vi "EventLog.Buffer.vi"(7 "action (get)":T7=enum."get", 8 "error in":errorcluster, 9 "Event.Sets":T5 {"dtm_End" format="%<%.1X\n%x>T"; "dtm_Begin" format="%<%.1X\n%x>T"}, 10 "Event in":T1={"ts"=0.0, "lev"=enum."Debug", "src"=enum."All", "msg"=enum."Log out", "arg"=[], "msg_str"=""} {"ts" format="%<%X\n%x>T"}, 11 "Translations":string[](array[string])) -> (0 "error out":errorcluster, 1 "Translated Msg":string, 2 "data out":T1[](array[typedef]) {"ts" format="%<%X\n%x>T"}, 3 "Event out":T1={"ts"=0.0, "lev"=enum."Debug", "src"=enum."All", "msg"=enum."Log out", "arg"=[], "msg_str"=""} {"ts" format="%<%X\n%x>T"})   [LabVIEW 2016]
uses:
  EventLog.Buffer.Action.ctl
  EventLog.EventGui.ctl
  EventLog.EventLevel.ctl
  EventLog.EventSource.ctl
  Translator/Translator.Message.ctl
  EventLog.Gui.Sets.ctl
  EventLog.EventLevelOperatorGui.ctl
panel:
  out "Translations out":string[](array[string])
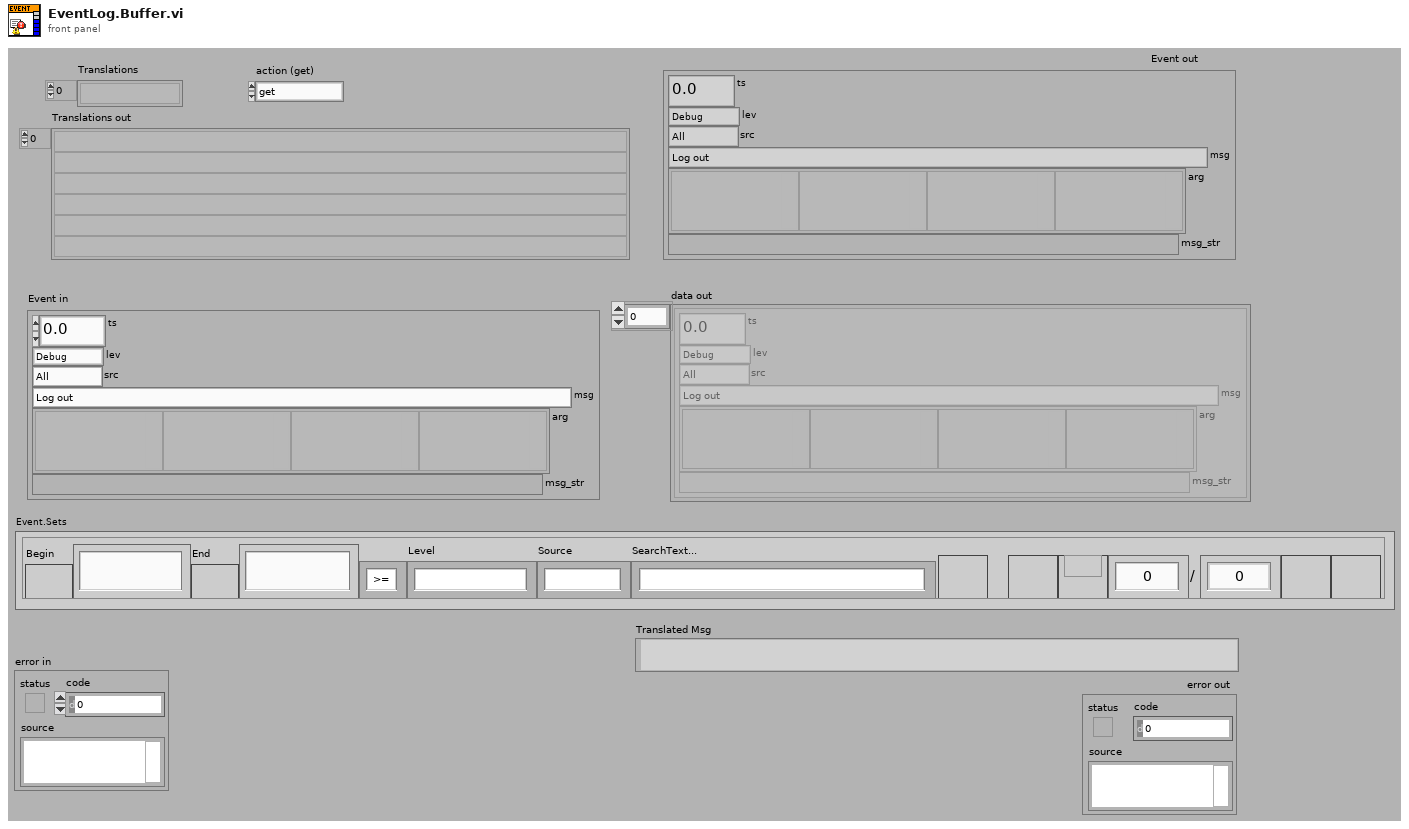
[diagram p1: front panel]
types:
  T1 = typedef "EventLog.EventGui.ctl" = cluster{"ts":dbl, "lev":T2, "src":T3, "msg":T4, "arg":variant[], "msg_str":string}
  T2 = typedef "EventLog.EventLevel.ctl" = enum8{"Debug", "Info", "Warning", "Error"}
  T3 = typedef "EventLog.EventSource.ctl" = enum16{"All", "Gui", "Cache", "PLC1", "PLC2", "PLC3", "DB", "DB01", "DB02", "DB03", "DB04", "DB05", "DB06", "DB07", "DB08", "DB09", "DB10", "DB11", "DB12", "DB13", "DB14", "DB15", "DB16"}
  T4 = typedef "Translator.Message.ctl" = enum16{"-", "Event confirmed", "Log out", "Log in", "Shutdown", "Cancel", "Start", "Continue", "Stop", "On", "Off", "OK", "NOK", "NOK %s", "This", "Prev", "Home", "Work", "In progress...", "Missing", "Empty", "Hardware failure", "Initial", "Error %d >> %s", "Error %d >> %s >> %s", "Starting %s", "Quitting %s", "Configured", "Initializing", "Quitting", "Loading", "Running %s", "Stopped", "Summary", "Do you want to continue?", "Do you want to exit?", "Log out?", "System", "All", "IDLE", "Translating...%s", "Not found", "Alarm %s", "Run", "Skip", "Abort", "Repeat", "Please wait...", "Database disconnected", "Login to database successful", "Login to database failed: %d; %s", "Get process step data for %s", "Changeover off", "Changeover into %s", "Product %s | %s found in cache with status %d at previous station", "Product %s | %s found in database with status %d at previous station", "Product %s | %s not found in cache at previous station", "Product %s | %s not found in database at previous station", "Product %s | %s found in cache with status %d at this station (%d repetion)", "Product %s | %s found in database with status %d at this station (%d repetition)", "Product %s | %s not found in cache at this station", "Product %s | %s not found in database at this station", "Product %s | %s found in cache for component %s | %s", "Product %s | %s found in database for component %s | %s", "Product not found in cache for component %s | %s", "Product not found in database for component %s | %s", "Product %s | %s connected with component %s | %s (cache)", "Product %s | %s connected with component %s | %s (database)", "New data for %s | %s (cache)", "New data for %s | %s (database)", "File %s moved (cache)", "File %s deleted (cache)", "Msg %d >> %s", "PLC LifeBit Failure", "Reconnecting DB", "Reconnecting PLC", "Free disk space is below 1GB - contact technician", "Unable to check product status"}
  T5 = typedef "EventLog.Gui.Sets.ctl" = cluster{"IncludeBegin":bool, "dtm_Begin":timestamp, "IncludeEnd":bool, "dtm_End":timestamp, "Events Level Operator":T6, "Level":u16, "Source":u16, "SearchText":string, "Refresh":bool, "Pages":i32, "PageNo":i32, "First":bool, "Prev":bool, "Next":bool, "Last":bool}
  T6 = typedef "EventLog.EventLevelOperatorGui.ctl" = enum16{">=", "=", "<="}
  T7 = typedef "EventLog.Buffer.Action.ctl" = enum16{"init", "re-init", "clear", "set translator", "translate", "add", "get"}
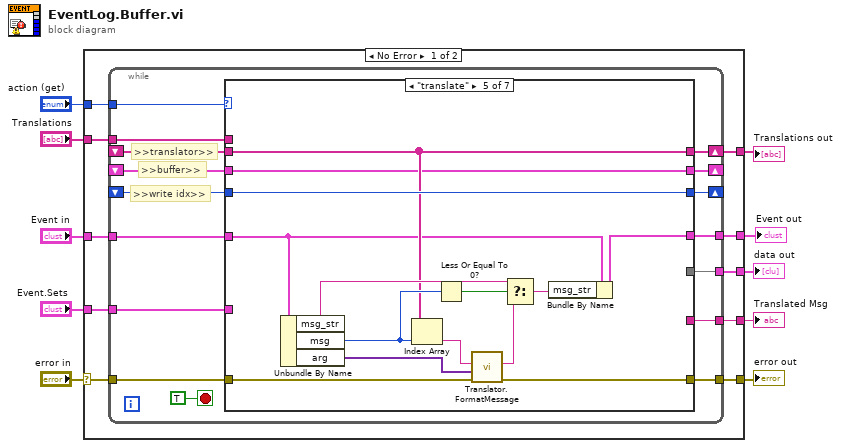
[diagram p0: block diagram]
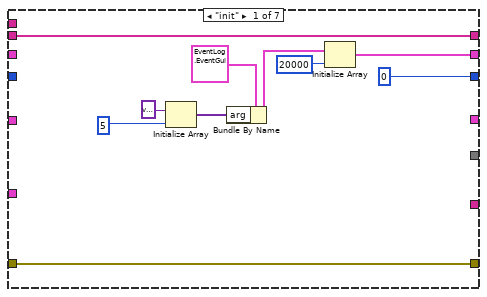
[diagram p2: hidden frame]
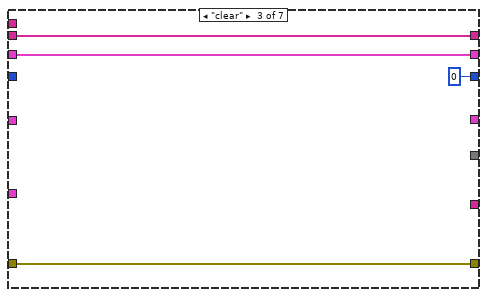
[diagram p4: hidden frame]
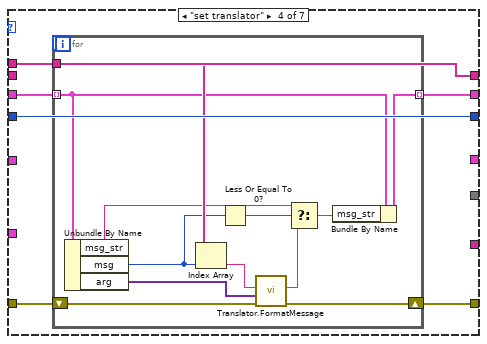
[diagram p5: hidden frame]
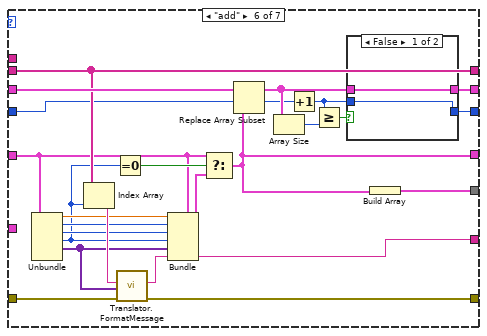
[diagram p6: hidden frame]
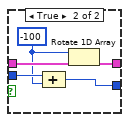
[diagram p7: hidden frame]
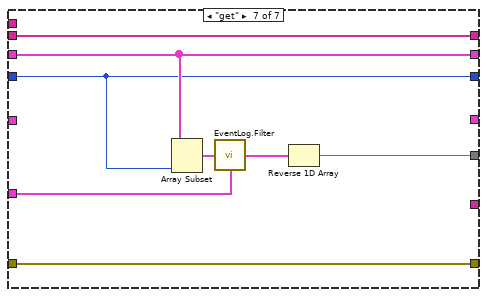
[diagram p8: hidden frame]
diagram:
  n1 = case shown="No Error" "error in" {
    selector: "error in" -> [w14 w125]
    tunnel: "action (get)" -> [w20 _]
    tunnel: "Event in" -> [w19 _]
    tunnel: [w18 _] -> w8
    tunnel: "Event.Sets" -> [w17 _]
    tunnel: "Translations" -> [w16 _]
    tunnel: [w15 w125] -> w6
    tunnel: [w13 _] -> w3
    tunnel: [w12 _] -> w2
    tunnel: [w11 _] -> w1
    frame No Error {
      n2 = while {
        tunnel: w20 -> [w35]
        tunnel: w19 -> [w34]
        shift-right: [w33] -> _
        shift-left: _ -> [w32]
        tunnel: [w31] -> w18
        shift-right: [w30] -> _
        shift-left: _ -> [w29]
        tunnel: w17 -> [w28]
        tunnel: w16 -> [w27]
        shift-right: [w26] -> w13
        shift-left: _ -> [w25]
        tunnel: w14 -> [w24]
        tunnel: [w23] -> w15
        tunnel: [w22] -> w12
        tunnel: [w21] -> w11
        stop <- TRUE stop-if-true
        # ">>write idx>>"
        # ">>translator>>"
        # ">>buffer>>"
        n3 = case shown="\"translate\"" w35 {
          tunnel: w34 -> [_ _ _ _ w74 w96 _]
          tunnel: [w45 w50 w54 w56 w75 w104 w118] -> w33
          tunnel: w32 -> [_ w50 w54 w59 w75 w109 w118]
          tunnel: [_ _ _ _ _ w98 w124] -> w31
          tunnel: [0 w49 0 w60 w86 w103 w117] -> w30
          tunnel: w29 -> [_ w49 _ w60 w86 w99 w117]
          tunnel: w28 -> [_ _ _ _ _ _ w122]
          tunnel: w27 -> [_ _ _ w55 _ _ _]
          tunnel: [w40 w48 w53 w55 w76 w101 w120] -> w26
          tunnel: w25 -> [w40 w48 w53 _ w76 w101 w120]
          tunnel: w24 -> [w38 w47 w52 w57 w84 w102 w119]
          tunnel: [w38 w47 w52 w58 w85 w91 w119] -> w23
          tunnel: [_ _ _ _ _ w87 _] -> w22
          tunnel: [_ _ _ _ w73 w90 _] -> w21
          frame "init" {
            n4 = Initialize Array(variant ("Variant"), 5 ("dimension size")) -> (w41:variant[])
            n5 = Bundle By Name(cluster=T1 {"ts"=0.0, "lev"=enum."Debug", "src"=enum."All", "msg"=enum."Log out", "arg"=[], "msg_str"=""} ("Event (GUI)"), "arg"=w41) -> (w44:T1)
            n6 = Initialize Array(w44, 20000 ("dimension size")) -> (w45:T1[])
          }
          frame "re-init" {
          }
          frame "clear" {
          }
          frame "set translator" {
            n7 = for {
              tunnel: w59 -> [w68] mode=indexing
              tunnel: w55 -> [w69]
              shift-right: [w71] -> w58
              shift-left: w57 -> [w70]
              tunnel: [w67] -> w56 mode=indexing
              n8 = Unbundle By Name(w68) -> ("msg_str"=w64:string, "msg"=w65:T4, "arg"=w72:variant[])
              n9 = Index Array(array=w69, index=w65) -> (element=w66:string)
              n10 = Less Or Equal To 0?(x=w65) -> (x <= 0?=w63:bool)
              n11 = call "Translator.FormatMessage.vi"("error in (no error)"=w70, "Arguments"=w72, "Msg"=w66) -> ("error out"=w71:errorcluster, "Translated Msg"=w62:string)  [unwired: 7 in]
              n12 = Select(t=w64, s=w63, f=w62) -> (s? t:f=w61:string)
              n13 = Bundle By Name(cluster=w68, "msg_str"=w61) -> (w67:T1)
            }
          }
          frame "translate" {
            n14 = Unbundle By Name(w74) -> ("msg_str"=w80:string, "msg"=w81:T4, "arg"=w83:variant[])
            n15 = Index Array(array=w76, index=w81) -> (element=w82:string)
            n16 = Less Or Equal To 0?(x=w81) -> (x <= 0?=w79:bool)
            n17 = call "Translator.FormatMessage.vi"("error in (no error)"=w84, "Arguments"=w83, "Msg"=w82) -> ("error out"=w85:errorcluster, "Translated Msg"=w78:string)  [unwired: 7 in]
            n18 = Select(t=w80, s=w79, f=w78) -> (s? t:f=w77:string)
            n19 = Bundle By Name(cluster=w74, "msg_str"=w77) -> (w73:T1)
          }
          frame "add" {
            n20 = Unbundle(w96) -> ("ts"=w94:dbl, "lev"=w93:T2, "src"=w92:T3, "msg"=w89:T4, "arg"=w88:variant[])  [unwired: 1 out]
            n21 = Index Array(array=w101, index=w89) -> (element=w100:string)
            n22 = Equal To 0?(x=w89) -> (x = 0?=w97:bool)
            n23 = call "Translator.FormatMessage.vi"("error in (no error)"=w102, "Arguments"=w88, "Msg"=w100) -> ("error out"=w91:errorcluster, "Translated Msg"=w87:string)  [unwired: 7 in]
            n24 = Bundle(cluster=w96, "ts"=w94, "lev"=w93, "src"=w92, "msg"=w89, "arg"=w88, "msg_str"=w87) -> (w95:T1)
            n25 = Select(t=w96, s=w97, f=w95) -> (s? t:f=w90:T1)
            n26 = Replace Array Subset(array=w109, new element=w90, index=w99) -> (w105:T1[])
            n27 = Array Size(array=w105) -> (size(s)=w108:i32)
            n28 = Increment(x=w99) -> (x+1=w106:i32)
            n29 = Greater Or Equal?(x=w106, y=w108) -> (x >= y?=w107:bool)
            n30 = case shown="False" w107 {
              tunnel: w106 -> [w110 w116]
              tunnel: w105 -> [w111 w115]
              tunnel: [w111 w114] -> w104
              tunnel: [w110 w112] -> w103
              frame False {
              }
              frame True {
                w113 = -100 ("y")
                n31 = Compound Arithmetic op=ADD(w116, w113) -> (w112:i32)
                n32 = Rotate 1D Array(1:w115, 2:w113) -> (0:w114:T1[])
              }
            }
            n33 = Build Array(w90) -> (w98:T1[])
          }
          frame "get" {
            n34 = Array Subset(array=w118, length=w117) -> (w123:T1[])  [unwired: 1 in]
            n35 = call "EventLog.Filter.vi"("data in"=w123, "Event.Sets"=w122) -> ("data out"=w121:T1[])
            n36 = Reverse 1D Array(array=w121) -> (reversed array=w124:T1[])
          }
        }
      }
    }
    frame Error {
    }
  }
  "error out" <- w6
  "data out" <- w8
  "Translations out" <- w3
  "Translated Msg" <- w2
  "Event out" <- w1
